vi "Publish.vi"(6 "Message ID":u16=10 format="%x", 7 "Publish Meta":T1, 8 "error in (no error)":errorcluster, 9 "Message to be published":string=" Message", 10 "Topic":string="a/b", 11 "connection ID":refnum<k5>) -> (0 "error out":errorcluster, 3 "connection ID out":refnum<k5>)   [LabVIEW 2020, in "DAQIO MQTT.lvlib"]
doc: "This VI publishes a message to a registered topic.\n\n© 2015 - daq.io, LLC - Peter Adelhardt"
uses:
  DAQIO MQTT.lvlib
  Controls/MessageType.ctl
  Controls/Publish Metadata.ctl
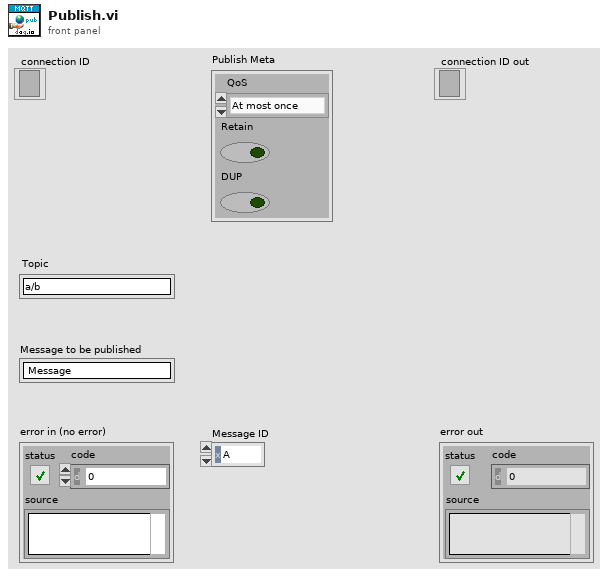
[diagram p1: front panel]
types:
  T1 = typedef "DAQIO MQTT.lvlib/Publish Metadata.ctl" = cluster{"QoS":enum8{"At most once", "At least once", "Exactly once", "Reserved"}, "Retain":bool, "DUP":bool}
  T2 = typedef "DAQIO MQTT.lvlib/MessageType.ctl" = enum32{"Reserved", "CONNECT", "CONNACK", "PUBLISH", "PUBACK", "PUBREC", "PUBREL", "PUBCOMP", "SUBSCRIBE", "SUBACK", "UNSUBSCRIBE", "UNSUBACK", "PINGREQ", "PINGRESP", "DISCONNECT", "Reserved2"}
  T3 = enum8{"At most once", "At least once", "Exactly once", "Reserved"}
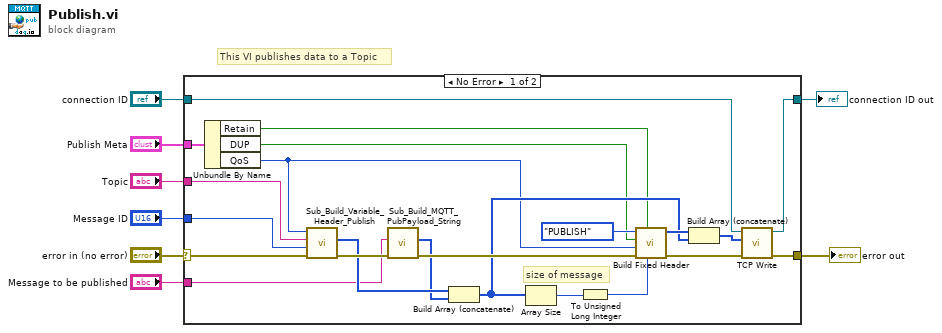
[diagram p0: block diagram]
diagram:
  # "This VI publishes data to a Topic"
  n1 = case shown="No Error" "error in (no error)" {
    selector: "error in (no error)" -> [w30 w32]
    tunnel: [w16 w32] -> w7
    tunnel: "Message to be published" -> [w15 _]
    tunnel: "Message ID" -> [w14 _]
    tunnel: "Publish Meta" -> [w13 _]
    tunnel: "Topic" -> [w12 _]
    tunnel: "connection ID" -> [w11 w31]
    tunnel: [w10 w31] -> w1
    frame No Error {
      # "size of message"
      n2 = Unbundle By Name(w13) -> ("Retain"=w20:bool, "DUP"=w19:bool, "QoS"=w9:T3)
      n3 = call "Sub_Build_Variable_Header_Publish.vi"("error in (no error)"=w30, "Message ID"=w14, "Topic Name"=w12, "QoS"=w9) -> ("error out"=w26:errorcluster, "Variable Header"=w24:u8[])  [unwired: 6 in]
      n4 = call "Sub_Build_MQTT_PubPayload_String.vi"("error in (no error)"=w26, "String to be encoded"=w15) -> ("error out"=w25:errorcluster, "UTF8 Byte Array"=w23:u8[])  [unwired: 8 in]
      n5 = Build Array (concatenate)(w24, w23) -> (w21:u8[])
      n6 = Array Size(array=w21) -> (size(s)=w27:i32)
      n7 = To Unsigned Long Integer(number=w27) -> (unsigned 32bit integer=w28:u32)
      n8 = call "Build Fixed Header.vi"("Remaining Length"=w28, "Retain"=w20, "error in (no error)"=w25, "QoS"=w9, "DUP"=w19, "MessageType"=MessageType."PUBLISH") -> ("error out"=w18:errorcluster, "Fixed Header"=w22:u8[])  [unwired: 4 in]
      n9 = Build Array (concatenate)(w22, w21) -> (w17:u8[])
      n10 = call "TCP Write.vi"("error in (no error)"=w18, "data in"=w17, "connection ID"=w11) -> ("error out"=w16:errorcluster, "connection ID out"=w10:refnum<k5>)  [unwired: 6 in, 1 out]
    }
    frame Error {
    }
  }
  "error out" <- w7
  "connection ID out" <- w1
